vi "SerializeMessage.vi"(7 "MsgSerializer":refnum<class "MsgSerializer.lvclass">, 9 "error in (no error)":errorcluster, 10 "Value":variant, 11 "TestManagerMsg.KVP in":refnum<class "TestManagerMsg.KVP.lvclass">) -> (1 "error out":errorcluster, 3 "Serialized Message":string)   [LabVIEW 2020, in "Caraya.lvlib" / "TestManagerMsg.KVP.lvclass"]
uses:
  TestManagerMsg.KVP.lvclass
  TestManagerMsg.KVP.lvclass/TestManagerMsg.KVP.ctl
  Test Manager Message/TestManagerMsg.lvclass
  <userlib>/_OpenG.lib/lvdata/lvdata.llb/openg_variant.lvlib
  C:/projects/caraya/src/classes/Test Manager Message/TestManagerMsg.lvclass
  MsgSerializer/MsgSerializer.lvclass
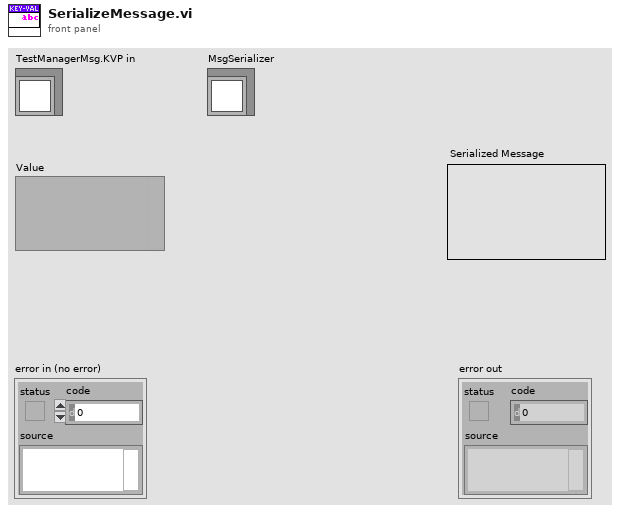
[diagram p1: front panel]
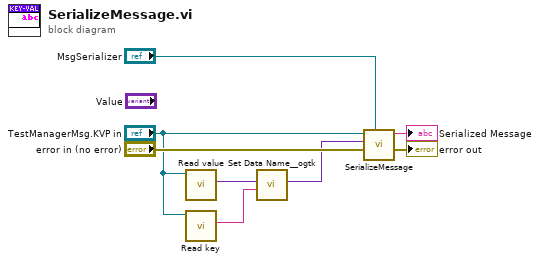
[diagram p0: block diagram]
diagram:
  n1 = call "Read value.vi"("TestManagerMsg.KVP in"="TestManagerMsg.KVP in") -> ("value"=w3:variant)  [unwired: 9 in, 1 out]
  n2 = call "Read key.vi"("TestManagerMsg in"="TestManagerMsg.KVP in") -> ("key"=w2:string)  [unwired: 9 in, 1 out]
  n3 = call <userlib>:"Set Data Name__ogtk.vi"("Data Name"=w2, "Data"=w3) -> ("Renamed Data"=w1:variant)  [unwired: 8 in, 1 out]
  n4 = call-parent "SerializeMessage.vi"("MsgSerializer"="MsgSerializer", "error in (no error)"="error in (no error)", "Value"=w1, "TestManagerMsg in"="TestManagerMsg.KVP in") -> ("error out"=→"error out":errorcluster, "Serialized Message"=→"Serialized Message":string)  [unwired: 6 in]
